vi "Set SpeedLimit(KB_s).vi"(8 "error in (no error)":errorcluster, 10 "SpeedLimit(KB/s)":i32, 11 "FileTransferOptions in":refnum<class "FileTransferOptions.lvclass">) -> (0 "error out":errorcluster, 3 "FileTransferOptions out":refnum<class "FileTransferOptions.lvclass">)   [LabVIEW 2015, in "WinSCP.lvlib" / "FileTransferOptions.lvclass"]
uses:
  FileTransferOptions.lvclass
  FileTransferOptions.lvclass/FileTransferOptions.ctl
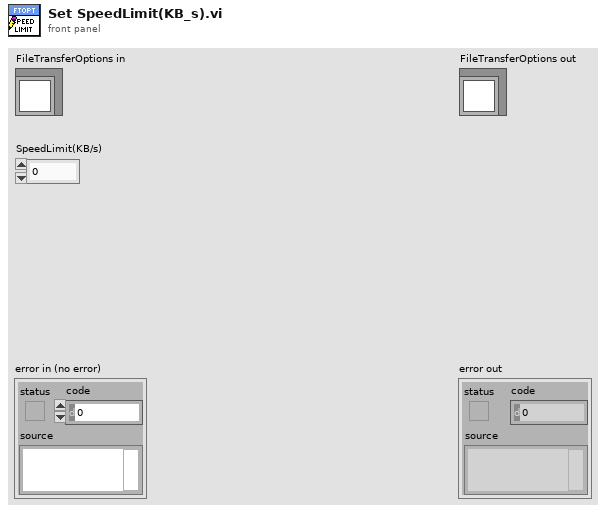
[diagram p1: front panel]
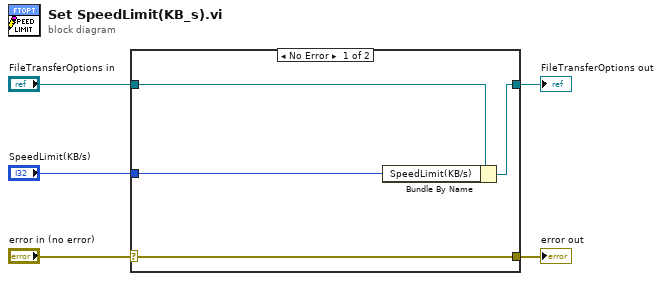
[diagram p0: block diagram]
diagram:
  n1 = case shown="No Error" "error in (no error)" {
    selector: "error in (no error)" -> [w9 w10]
    tunnel: [w9 w10] -> w4
    tunnel: [w7 w11] -> w2
    tunnel: "FileTransferOptions in" -> [w8 w11]
    tunnel: "SpeedLimit(KB/s)" -> [w6 _]
    frame No Error {
      n2 = Bundle By Name(cluster=w8, "SpeedLimit(KB/s)"=w6) -> (w7:refnum<class "FileTransferOptions.lvclass">)
    }
    frame Error {
    }
  }
  "error out" <- w4
  "FileTransferOptions out" <- w2
